vi "ReadButtonBar.vi"(8 "Error In":errorcluster, 11 "reference in":refnum<class "VerticalButtonBar.lvclass">) -> (0 "Error Out":errorcluster, 2 "ButtonBar":refnum<class "ButtonCollection.lvclass"> caption="Object Out", 3 "reference in":refnum<class "VerticalButtonBar.lvclass">)   [LabVIEW 2021, in "VerticalButtonBar.lvclass"]
uses:
  VerticalButtonBar.lvclass
  ButtonCollection/ButtonCollection.lvclass
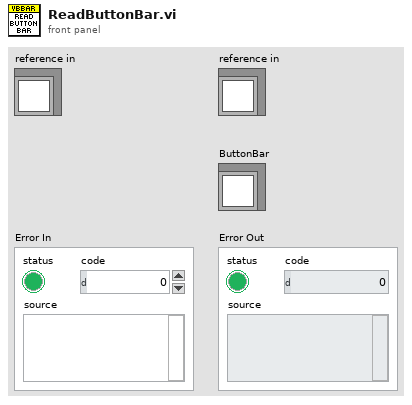
[diagram p1: front panel]
types:
  T1 = typedef "VerticalButtonBar.lvclass/ObjectAttributes.ctl" = cluster{"Interfaces":cluster{"IDockGUI":refnum<class "IDockGUI.lvclass">, "Authorizer":refnum<class "IAuthorization.lvclass">}, "Locals":cluster{"ButtonBar":refnum<class "ButtonCollection.lvclass">, "BaseConfigurationPath":path, "Labels":cluster{"Label":string, "Value":string}[]}, "Persistent":cluster{"ButtonDefinitionFile":string}}
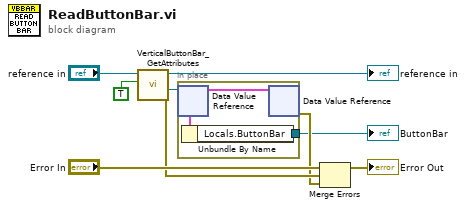
[diagram p0: block diagram]
diagram:
  n1 = call "VerticalButtonBar_GetAttributes.vi"("OnlyGetDvrReference(False)"=TRUE, "reference in"="reference in") -> ("error out"=w6:errorcluster, "DataRef"=w3:refnum<data-value>, "reference out"=→"reference in":refnum<class "VerticalButtonBar.lvclass">)  [unwired: 6 in, 1 out]
  n2 = in-place {
    in-place-border: [w11] -> w1
    n3 = in-place-dvr #1(w3) -> (w10:T1)  [unwired: 1 out]
    n4 = Unbundle By Name(w10) -> ("Locals.ButtonBar"=w11:refnum<class "ButtonCollection.lvclass">)
    n5 = in-place-dvr #1(w10) -> (w2:errorcluster)  [unwired: 1 out]
  }
  "ButtonBar" <- w1
  n6 = Merge Errors("Error In", w6, w2) -> (→"Error Out":errorcluster)
